vi "flush DAQ buffer.vi"(8 "error in":errorcluster, 11 "App Data":T1) -> (0 "error out":errorcluster)   [LabVIEW 2014]
uses:
  Controls/App Data.ctl
  <vilib>/DAQmx/read.llb/DAQmx Read (Analog 2D DBL NChan NSamp).vi
  <vilib>/DAQmx/miscellaneous.llb/DAQmx Fill In Error Info.vi
  <resource>/objmgr/daqmx.rc
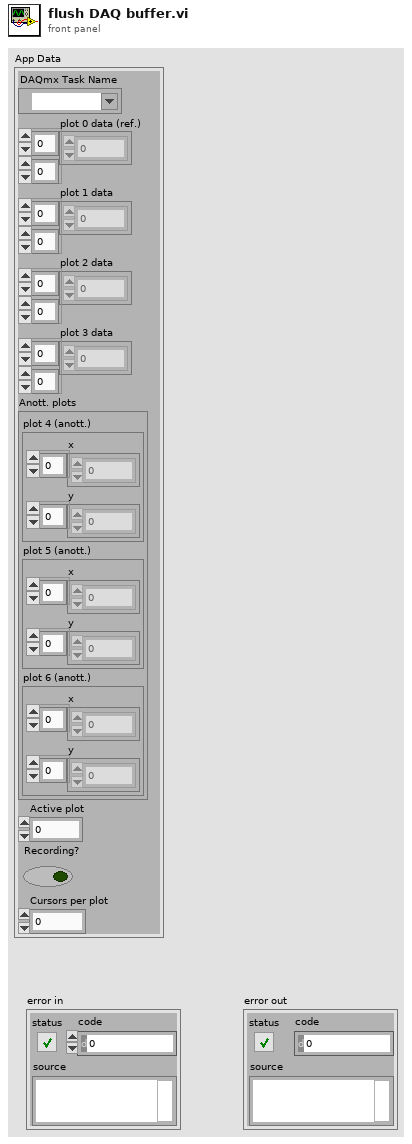
[diagram p1: front panel]
types:
  T1 = typedef "App Data.ctl" = cluster{"DAQmx Task Name":refnum<k21>, "plot 0 data (ref.)":dbl[][], "plot 1 data":dbl[][], "plot 2 data":dbl[][], "plot 3 data":dbl[][], "Anott. plots":cluster{"plot 4 (anott.)":cluster{"x":dbl[], "y":dbl[]}, "plot 5 (anott.)":cluster{"x":dbl[], "y":dbl[]}, "plot 6 (anott.)":cluster{"x":dbl[], "y":dbl[]}}, "Active plot":u32, "Recording?":bool, "Cursors per plot":i32}
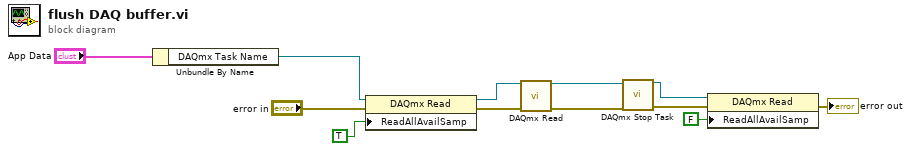
[diagram p0: block diagram]
diagram:
  n1 = Unbundle By Name("App Data") -> ("DAQmx Task Name"=w3:refnum<k21>)
  n2 = property class="DAQmx Read"(reference=w3, error in="error in", "ReadAllAvailSamp"=TRUE) -> (reference out=w10:refnum<k21>, error out=w8:errorcluster)
  n3 = call-poly <vilib>:"DAQmx Read.vi"("task/channels in"=w10, "error in"=w8) -> ("task out"=w9:refnum<k21>, "error out"=w12:errorcluster)  [unwired: 11 in, 1 out]
  n4 = call <vilib>:"DAQmx Stop Task.vi"("task/channels in"=w9, "error in"=w12) -> ("task out"=w5:refnum<k21>, "error out"=w6:errorcluster)  [unwired: 12 in]
  n5 = property class="DAQmx Read"(reference=w5, error in=w6, "ReadAllAvailSamp"=FALSE) -> (error out=→"error out":errorcluster)  [unwired: 1 out]
